vi "Configure_HW_dialog.vi"() -> (3 "output":T1={"SQUID"={"port"="", "Flux constant"={"X"=8.34e-05, "Y"=-8.11e-05, "Z"=-4.28e-05}, "X"=10, "Y"=10, "Z"=10}, "Sample Handler"={"port"="", "BG 1"=-82132, "BG 2"=-22571, "Sensor"=-74765, "AF 1"=-51160, "AF 2"=-123198, "AF coil"=-110030, "Home (absolute)"=0, "Home (relative to limit switch)"=989, "robot"=40750}, "Degausser"={"port"="", "Tracking timeout (sec)"=60, "Communication Delays"=350}, "ARM Unit"={"port"=""}, "IRM Unit（未実装）"={"port"=""}, "Robot"={"port"=""}} {"SQUID"."Z" items=["1 Hz"=1, "10 Hz"=10, "100 Hz"=100, "WB"=0]; "SQUID"."Y" items=["1 Hz"=1, "10 Hz"=10, "100 Hz"=100, "WB"=0]; "SQUID"."X" items=["1 Hz"=1, "10 Hz"=10, "100 Hz"=100, "WB"=0]})   [LabVIEW 2017]
doc: "イベント処理を使用するダイアログボックスを作成するのにこのテンプレートを使用します。"
uses:
  controls/HW Configuration.ctl
  controls/SQUID_configuration.ctl
  controls/XYZ_Data.ctl
  controls/SQUID_filter.ctl
  controls/SampleHandler_configuration.ctl
  controls/Degausser_configuration.ctl
  <vilib>/Utility/xml.llb/Write to XML File(string).vi
  <vilib>/Utility/xml.llb/Read From XML File(string).vi
panel:
  in  "Save as":bool
  in  "Load":bool
  in  "Hardware":T1={"SQUID"={"port"="COM9", "Flux constant"={"X"=8.34e-05, "Y"=-8.11e-05, "Z"=-4.28e-05}, "X"=10, "Y"=10, "Z"=10}, "Sample Handler"={"port"="COM7", "BG 1"=82132, "BG 2"=22571, "Sensor"=74765, "AF 1"=51160, "AF 2"=123198, "AF coil"=110030, "Home (absolute)"=0, "Home (relative to limit switch)"=989, "robot"=40750}, "Degausser"={"port"="COM10", "Tracking timeout (sec)"=60, "Communication Delays"=350}, "ARM Unit"={"port"="COM8"}, "IRM Unit（未実装）"={"port"=""}, "Robot"={"port"="TCPIP0::192.168.0.20::2000::SOCKET"}} {"SQUID"."Z" items=["1 Hz"=1, "10 Hz"=10, "100 Hz"=100, "WB"=0]; "SQUID"."Y" items=["1 Hz"=1, "10 Hz"=10, "100 Hz"=100, "WB"=0]; "SQUID"."X" items=["1 Hz"=1, "10 Hz"=10, "100 Hz"=100, "WB"=0]}
  in  "Cancel":bool caption="キャンセル"
  in  "OK":bool
  # "Count (Positive=RH)"
  # "Relative to Home?"
  # "Filter (未実装）"
  # "Count (Positive=RH)"
  # "Relative to Home?"
  # "Filter (未実装）"
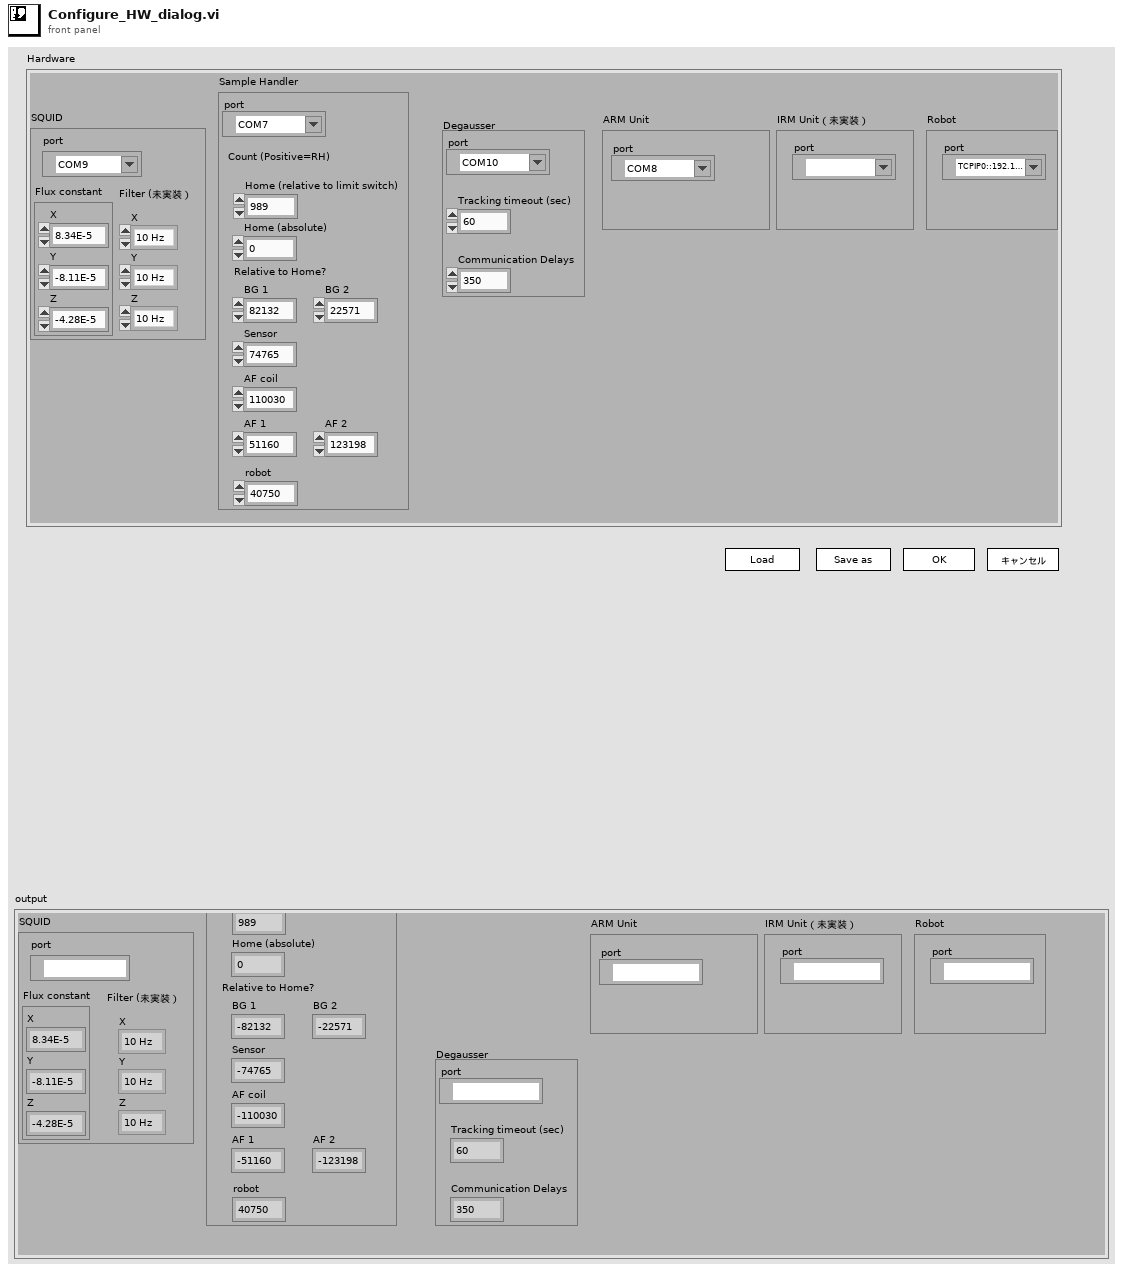
[diagram p1: front panel]
types:
  T1 = typedef "HW Configuration.ctl" = cluster{"SQUID":T2, "Sample Handler":T5, "Degausser":T6, "ARM Unit":cluster{"port":refnum<visa-resource-name>}, "IRM Unit（未実装）":cluster{"port":refnum<visa-resource-name>}, "Robot":cluster{"port":refnum<visa-resource-name>}}
  T2 = typedef "SQUID_configuration.ctl" = cluster{"port":refnum<visa-resource-name>, "Flux constant":T3, "X":T4, "Y":T4, "Z":T4}
  T3 = typedef "XYZ_Data.ctl" = cluster{"X":dbl, "Y":dbl, "Z":dbl}
  T4 = typedef "SQUID_filter.ctl" = u16
  T5 = typedef "SampleHandler_configuration.ctl" = cluster{"port":refnum<visa-resource-name>, "BG 1":i32, "BG 2":i32, "Sensor":i32, "AF 1":i32, "AF 2":i32, "AF coil":i32, "Home (absolute)":i32, "Home (relative to limit switch)":i32, "robot":i32}
  T6 = typedef "Degausser_configuration.ctl" = cluster{"port":refnum<visa-resource-name>, "Tracking timeout (sec)":i16, "Communication Delays":i16}
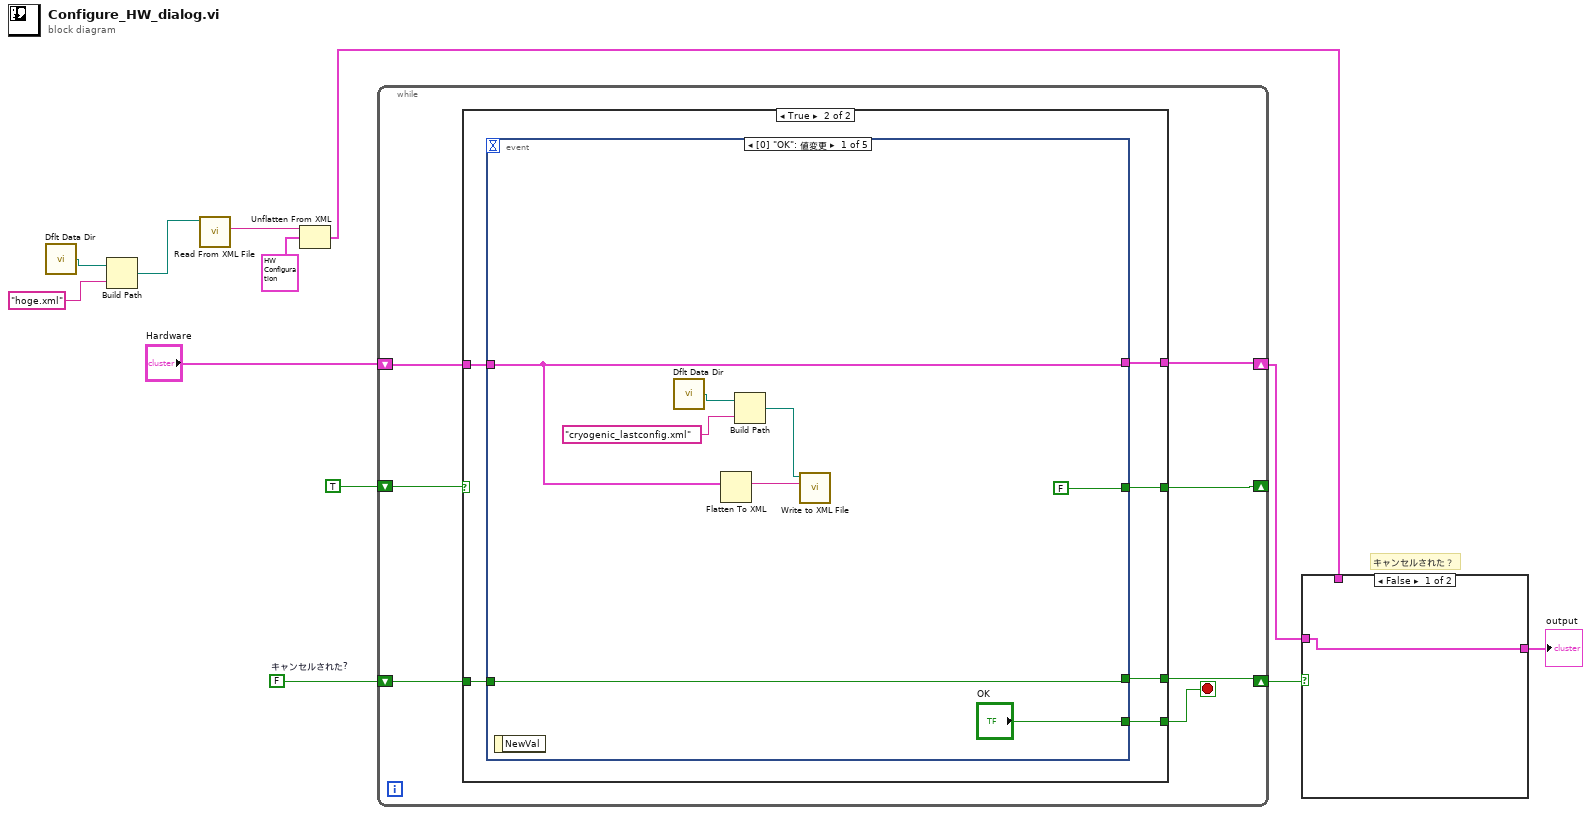
[diagram p0: block diagram]
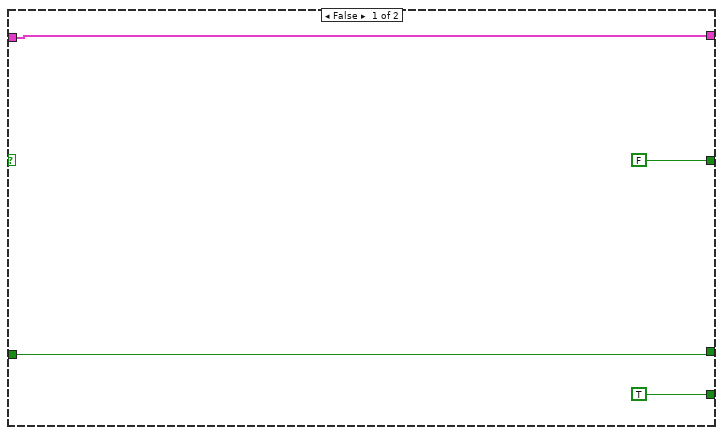
[diagram p3: hidden frame]
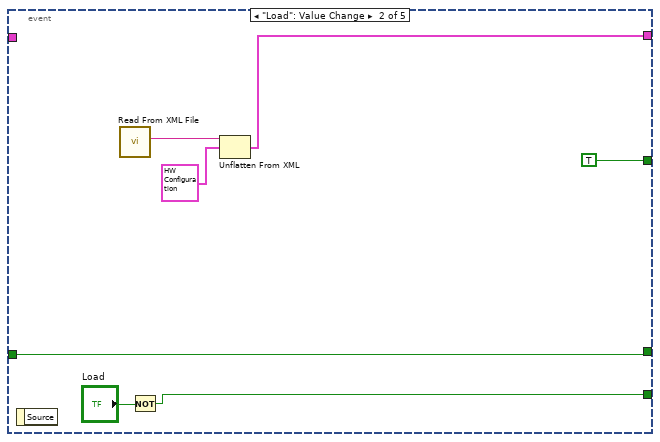
[diagram p4: hidden frame]
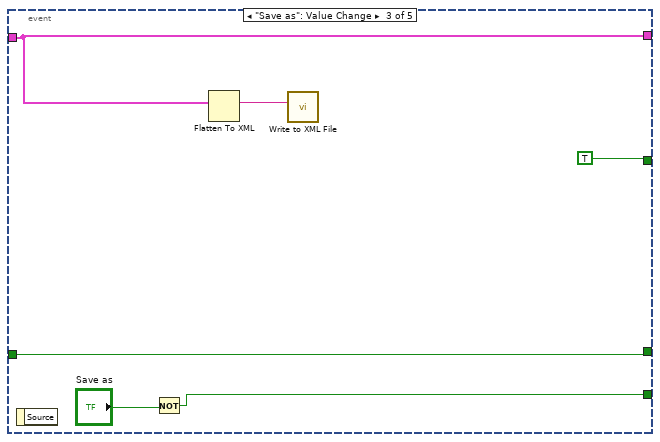
[diagram p5: hidden frame]
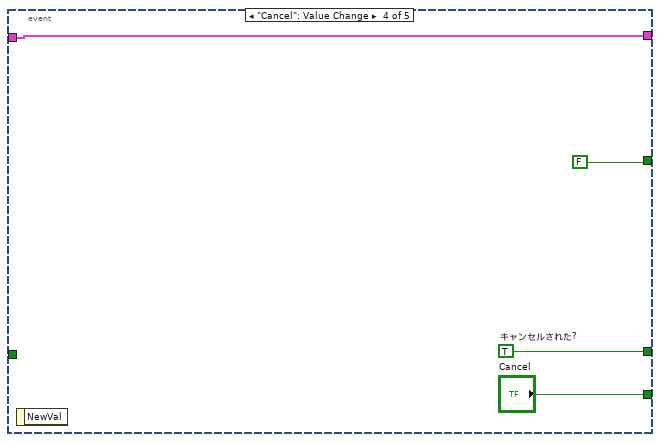
[diagram p6: hidden frame]
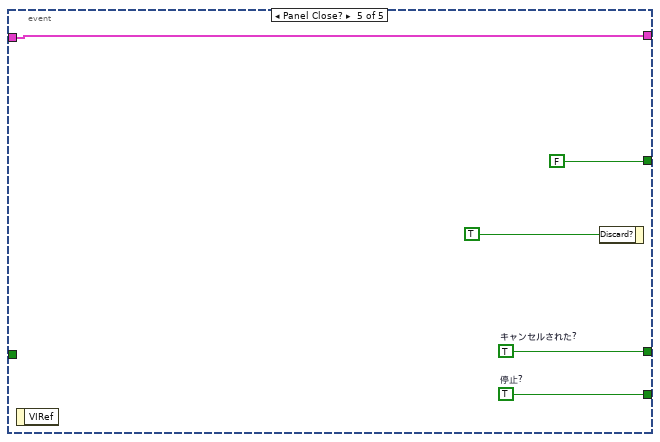
[diagram p7: hidden frame]
diagram:
  w11 = FALSE  # キャンセルされた?
  # "キャンセルされた？"
  n1 = call <vilib>:"Dflt Data Dir.vi"() -> ("App:Default Data Directory"=w3:path)
  n2 = Build Path(base path=w3, name or relative path="hoge.xml") -> (appended path=w1:path)
  n3 = call-poly <vilib>:"Read From XML File.vi"("XML File Path"=w1) -> ("XML Elements"=w5:string)  [unwired: 8 in, 2 out]
  n4 = Unflatten From XML(xml string=w5, type=T1 {"SQUID"={"port"="", "Flux constant"={"X"=8.34e-05, "Y"=-8.11e-05, "Z"=-4.28e-05}, "X"=10, "Y"=10, "Z"=10}, "Sample Handler"={"port"="", "BG 1"=-82132, "BG 2"=-22571, "Sensor"=-74765, "AF 1"=-51160, "AF 2"=-123198, "AF coil"=-110030, "Home (absolute)"=0, "Home (relative to limit switch)"=989, "robot"=40750}, "Degausser"={"port"="", "Tracking timeout (sec)"=60, "Communication Delays"=350}, "ARM Unit"={"port"=""}, "IRM Unit（未実装）"={"port"=""}, "Robot"={"port"=""}} ("Hardware")) -> (value=w7:T1)  [unwired: 1 in, 1 out]
  n5 = while {
    shift-right: [w16] -> _
    shift-left: TRUE -> [w14]
    shift-right: [w18] -> w10
    shift-left: w11 -> [w15]
    shift-right: [w13] -> w8
    shift-left: "Hardware" -> [w17]
    stop <- w19 stop-if-true
    n6 = case shown="TRUE" w14 {
      tunnel: [TRUE w29] -> w19
      tunnel: [w21 w25] -> w18
      tunnel: w17 -> [w20 w28]
      tunnel: [FALSE w27] -> w16
      tunnel: w15 -> [w21 w26]
      tunnel: [w20 w24] -> w13
      frame False {
      }
      frame True {
        n7 = event shown="[0] \"OK\": 値変更" {
          selector: _ -> [_ _ _ _ _]
          dyn-events: _ -> [_ _ _ _ _]
          timeout: _ -> [_ _ _ _ _]
          tunnel: ["OK" w41 w46 "Cancel" w58] -> w29
          tunnel: [w35 w43 w48 w54 w57] -> w25
          tunnel: w28 -> [w33 _ w45 w51 w55]
          tunnel: [FALSE TRUE TRUE FALSE FALSE] -> w27
          tunnel: w26 -> [w35 w43 w48 _ _]
          tunnel: [w33 w38 w45 w51 w55] -> w24
          event "OK": Value Change {
            n8 = event-data() -> ()  [unwired: 1 in, 1 out]
            n9 = call <vilib>:"Dflt Data Dir.vi"() -> ("App:Default Data Directory"=w32:path)
            n10 = Flatten To XML(anything=w33) -> (xml string=w34:string)
            n11 = Build Path(base path=w32, name or relative path="cryogenic_lastconfig.xml") -> (appended path=w30:path)
            n12 = call-poly <vilib>:"Write to XML File.vi"("XML Input"=w34, "XML File Path"=w30) -> ()  [unwired: 7 in, 3 out]
          }
          event "Load": Value Change {
            n13 = event-data() -> ()  [unwired: 1 in, 1 out]
            n14 = call-poly <vilib>:"Read From XML File.vi"() -> ("XML Elements"=w40:string)  [unwired: 9 in, 2 out]
            n15 = Not(x="Load") -> (.not. x?=w41:bool)
            n16 = Unflatten From XML(xml string=w40, type=T1 {"SQUID"={"port"="", "Flux constant"={"X"=8.34e-05, "Y"=-8.11e-05, "Z"=-4.28e-05}, "X"=10, "Y"=10, "Z"=10}, "Sample Handler"={"port"="", "BG 1"=-82132, "BG 2"=-22571, "Sensor"=-74765, "AF 1"=-51160, "AF 2"=-123198, "AF coil"=-110030, "Home (absolute)"=0, "Home (relative to limit switch)"=989, "robot"=40750}, "Degausser"={"port"="", "Tracking timeout (sec)"=60, "Communication Delays"=350}, "ARM Unit"={"port"=""}, "IRM Unit（未実装）"={"port"=""}, "Robot"={"port"=""}} ("Hardware")) -> (value=w38:T1)  [unwired: 1 in, 1 out]
          }
          event "Save as": Value Change {
            n17 = event-data() -> ()  [unwired: 1 in, 1 out]
            n18 = Not(x="Save as") -> (.not. x?=w46:bool)
            n19 = Flatten To XML(anything=w45) -> (xml string=w50:string)
            n20 = call-poly <vilib>:"Write to XML File.vi"("XML Input"=w50) -> ()  [unwired: 8 in, 3 out]
          }
          event "Cancel": Value Change {
            w54 = TRUE  # キャンセルされた?
            n21 = event-data() -> ()  [unwired: 1 in, 1 out]
          }
          event Panel Close? {
            w57 = TRUE  # キャンセルされた?
            w58 = TRUE  # 停止?
            n22 = event-data() -> ()  [unwired: 1 in, 1 out]
            n23 = event-data("Discard?"=TRUE) -> ()  [unwired: 1 in, 1 out]
          }
        }
      }
    }
  }
  n24 = case shown="FALSE" w10 {
    tunnel: w7 -> [_ w61]
    tunnel: [w60 w61] -> w9
    tunnel: w8 -> [w60 _]
    frame False {
    }
    frame True {
    }
  }
  "output" <- w9
